vi "ConfigUtilities - Initialize Main Page Panel.vi"(8 "error in (no error)":errorcluster, 10 "Main Page References":T1, 11 "Item Ref in":T2 format="%.0x") -> (0 "error out":errorcluster, 3 "Item Ref out":T2 format="%.0x")   [LabVIEW 2015, in "UDP-Custom-Device System Explorer.lvlib"]
doc: "Initializes the Main Page front panel from the properties."
uses:
  UDP-Custom-Device System Explorer.lvlib
  <vilib>/NI Veristand/Custom Device API/Custom Device Item Ref.ctl
  Types/UDP Data Link - TypeDefs - Main Page References.ctl
  Shared/Constants.vi
  <vilib>/NI Veristand/Custom Device API/Get Item Property (Dependent Node Pointer).vi
  <vilib>/NI VeriStand/Custom Device API/Custom Device API.lvlib
  Shared/UDP-Custom-Device Shared.lvlib
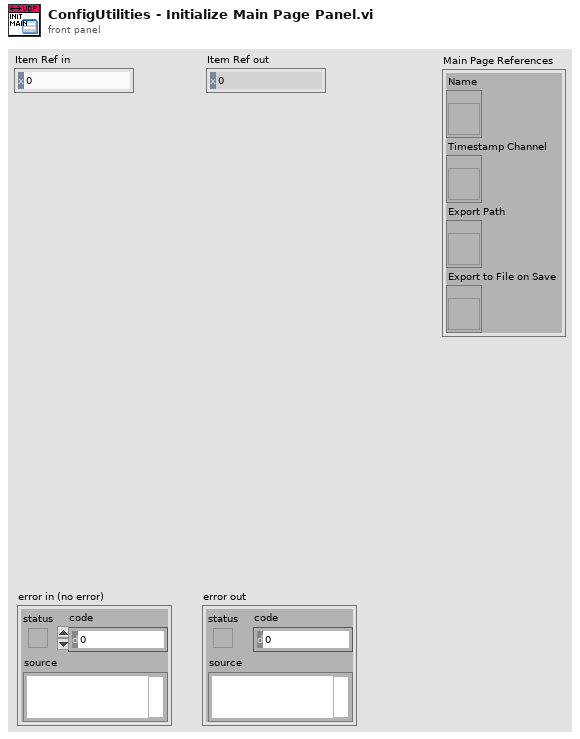
[diagram p1: front panel]
types:
  T1 = typedef "UDP-Custom-Device System Explorer.lvlib/UDP Data Link - TypeDefs - Main Page References.ctl" = cluster{"Name":refnum<vi>, "Timestamp Channel":refnum<vi>, "Export Path":refnum<vi>, "Export to File on Save":refnum<vi>}
  T2 = typedef "Custom Device API.lvlib/Custom Device Item Ref.ctl" = u64
  T3 = typedef "Custom Device API.lvlib/Custom Device Item Info.ctl" = cluster{"Name":string, "Is Channel":bool, "GUID":string, "Is Waveform":bool}
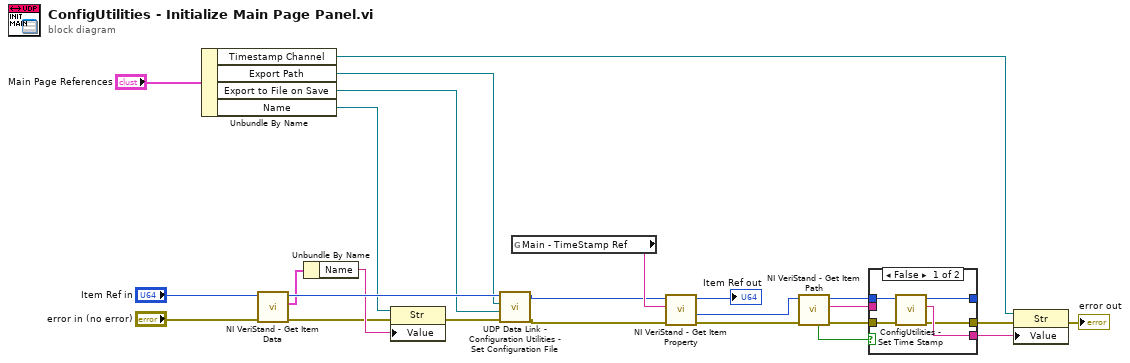
[diagram p0: block diagram]
diagram:
  n1 = Unbundle By Name("Main Page References") -> ("Timestamp Channel"=w3:refnum<vi>, "Export Path"=w7:refnum<vi>, "Export to File on Save"=w8:refnum<vi>, "Name"=w11:refnum<vi>)
  n2 = call <vilib>:"NI VeriStand - Get Item Data.vi"("error in (no error)"="error in (no error)", "Item Ref in"="Item Ref in") -> ("error out"=w10:errorcluster, "Item Info"=w13:T3, "Item Ref out"=w25:T2)  [unwired: 7 out]
  n3 = Unbundle By Name(w13) -> ("Name"=w14:string)
  n4 = property class="Str"(reference=w11, error in=w10, "Value"=w14) -> (error out=w9:errorcluster)  [unwired: 1 out]
  n5 = call "UDP Data Link - Configuration Utilities - Set Configuration File.vi"("error in (no error)"=w9, "Export to File on Save"=w8, "Export Path"=w7, "Item Ref in"=w25) -> ("error out"=w1:errorcluster, "Item Ref out"=w2:T2)  [unwired: 6 in]
  n6 = global read "Constants.vi" "Main - TimeStamp Ref"() -> (w4:string)
  n7 = call-poly <vilib>:"NI VeriStand - Get Item Property.vi"("error in (no error)"=w1, "Property Name"=w4, "Item Ref in"=w2) -> ("error out"=w18:errorcluster, "Dependent Node Ref"=w24:T2, "Item Ref out"=→"Item Ref out":T2)  [unwired: 5 in, 1 out]
  n8 = call <vilib>:"NI VeriStand - Get Item Path.vi"("error in (no error)"=w18, "Item Ref in"=w24) -> ("error out"=w22:errorcluster, "Path"=w20:string, "Item Ref out"=w21:T2, "Found"=w19:bool)  [unwired: 6 in]
  n9 = case shown="False" w19 {
    tunnel: w20 -> [_ w32]
    tunnel: w21 -> [w29 w33]
    tunnel: w22 -> [w30 w31]
    tunnel: [w28 w33] -> _
    tunnel: [w27 w32] -> w23
    tunnel: [w26 w31] -> w6
    frame False {
      n10 = call "ConfigUtilities - Set Time Stamp.vi"("error in (no error)"=w30, "Device Item Ref in"=w29) -> ("error out"=w26:errorcluster, "Path"=w27:string, "Device Item Ref out"=w28:T2)  [unwired: 7 in]
    }
    frame True {
    }
  }
  n11 = property class="Str"(reference=w3, error in=w6, "Value"=w23) -> (error out=→"error out":errorcluster)  [unwired: 1 out]
